vi "CreateConfigRegisters.vi"(0 "LimitsEnabled":u16, 5 "UnscaledHighLimit":i16[](array[numeric])=[0, 0, 0, 0, 0, 0, 0, 0, 0, 0, 0, 0, 0, 0, 0, 0], 7 "UnscaledLowLimit":i16[](array[numeric])=[0, 0, 0, 0, 0, 0, 0, 0, 0, 0, 0, 0, 0, 0, 0, 0], 9 "B":i16[](array[numeric])=[0, 0, 0, 0, 0, 0, 0, 0, 0, 0, 0, 0, 0, 0, 0, 0], 11 "M":sgl[](array[numeric])=[0.0, 0.0, 0.0, 0.0, 0.0, 0.0, 0.0, 0.0, 0.0, 0.0, 0.0, 0.0, 0.0, 0.0, 0.0, 0.0]) -> (4 "ConfigRegisters":T1)   [LabVIEW 2017, in "ScaleAndLimit.lvlib"]
doc: "Creates and initializes the scale and limits registers."
uses:
  ScaleAndLimit.lvlib
  ConfigRegisters.ctl
  <vilib>/rvi/DataTransferAndStorage/Container/Common/niFpgaContainerGetUniqueNameForEmu.vi
  <vilib>/rvi/DataTransferAndStorage/Container/Common/niFpgaContainerSetEmuInfo.vi
  <vilib>/rvi/eio/common/nirviEmuReportErrorAndStop.vi
  <vilib>/rvi/DataTransferAndStorage/Container/Common/niFpgaContainerExecOnDevCompGetState.vi
  <vilib>/rvi/Emulation/niFpgaEmulationIsFPGAContextNoSignature.vi
  <vilib>/rvi/Memory/Memory_Emulation/niFpgaMemoryEmulationCacheClearOnFirstRun.vi
  <vilib>/rvi/Memory/Memory_Emulation/nirvimemoryEmulationManagerCache_MakeExclusive.vi
  <vilib>/rvi/Memory/Memory_Emulation/niFpgaMemoryEmulationValidateCache.vi
  <vilib>/rvi/Memory/Memory_Emulation/nirvimemoryEmulationManagerCache_InsertValue.vi
  <vilib>/Utility/error.llb/Clear Errors.vi
  <vilib>/rvi/Memory/Memory_Emulation/nirvimemoryEmulationManagerCache_ReleaseExclusive.vi
  <vilib>/rvi/Memory/Memory_Emulation/nirvimemoryEmulationManagerCache_GetValue.vi
  <vilib>/rvi/Memory/Memory_Emulation/nirvimemoryEmulationManagerCache_SetValue.vi
  <vilib>/rvi/Emulation/niFpgaProcessEmulError.vi
  <vilib>/rvi/Emulation/niFpgaSctlEmulationGetInTimedLoop.vi
  <vilib>/rvi/LocalResourceManager/LocalResourceManager.xnode
  <vilib>/rvi/DataTransferAndStorage/Container/XNode/niFpgaContainer.xnode
  <vilib>/rvi/DataTransferAndStorage/Register/Emulation/niFpgaRegisterEmulationRefIn.vi
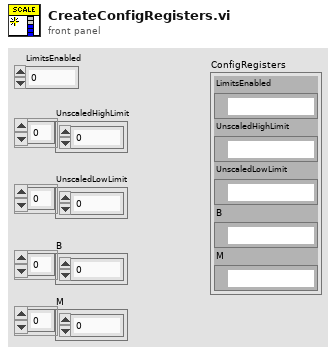
[diagram p1: front panel]
types:
  T1 = typedef "ScaleAndLimit.lvlib/ConfigRegisters.ctl" = cluster{"LimitsEnabled":refnum<k21>, "UnscaledHighLimit":refnum<k21>, "UnscaledLowLimit":refnum<k21>, "B":refnum<k21>, "M":refnum<k21>}
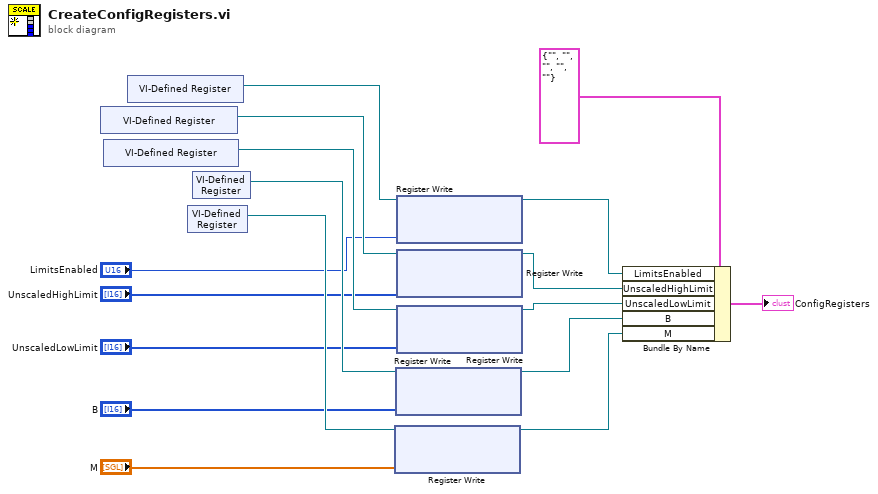
[diagram p0: block diagram]
diagram:
  n1 = xnode "VI-Defined Register"() -> ("Register Out"=w10:refnum<k21>)
  n2 = xnode "VI-Defined Register"() -> ("Register Out"=w12:refnum<k21>)
  n3 = xnode "VI-Defined Register"() -> ("Register Out"=w9:refnum<k21>)
  n4 = xnode "VI-Defined Register"() -> ("Register Out"=w16:refnum<k21>)
  n5 = xnode "VI-Defined Register"() -> ("Register Out"=w14:refnum<k21>)
  n6 = xnode "Register Write"("Data"="M", "Register In"=w16) -> ("Register Out"=w2:refnum<k21>)
  n7 = xnode "Register Write"("Data"="B", "Register In"=w14) -> ("Register Out"=w3:refnum<k21>)
  n8 = xnode "Register Write"("Data"="LimitsEnabled", "Register In"=w9) -> ("Register Out"=w6:refnum<k21>)
  n9 = xnode "Register Write"("Data"="UnscaledHighLimit", "Register In"=w10) -> ("Register Out"=w5:refnum<k21>)
  n10 = xnode "Register Write"("Data"="UnscaledLowLimit", "Register In"=w12) -> ("Register Out"=w4:refnum<k21>)
  n11 = Bundle By Name(cluster=T1 {"LimitsEnabled"="", "UnscaledHighLimit"="", "UnscaledLowLimit"="", "B"="", "M"=""} ("ConfigRegisters"), "LimitsEnabled"=w6, "UnscaledHighLimit"=w5, "UnscaledLowLimit"=w4, "B"=w3, "M"=w2) -> (→"ConfigRegisters":T1)
